vi "update execution error.vi"(8 "error in (no error)":errorcluster, 11 "Channel in":refnum<class "Channel.lvclass">) -> (0 "error out":errorcluster, 3 "Channel out":refnum<class "Channel.lvclass">)   [LabVIEW 2018, in "Channel.lvclass"]
doc: "Verify if there is an error in the error array of the camera class\n\nThis function will return true if there is any error or warning in the error array of the camera with a code different of 20002 or 0."
uses:
  Channel.lvclass
  Channel.lvclass/Channel.ctl
  Simulated_CCD_Camera/Simulated_CCD_Camera.lvclass/Simulated_CCD_Camera.ctl
  <vilib>/Utility/error.llb/Error Cluster From Error Code.vi
  <vilib>/ErrorRing/Error Ring.xnode
  Simulated_CCD_Camera/Simulated_CCD_Camera.lvclass
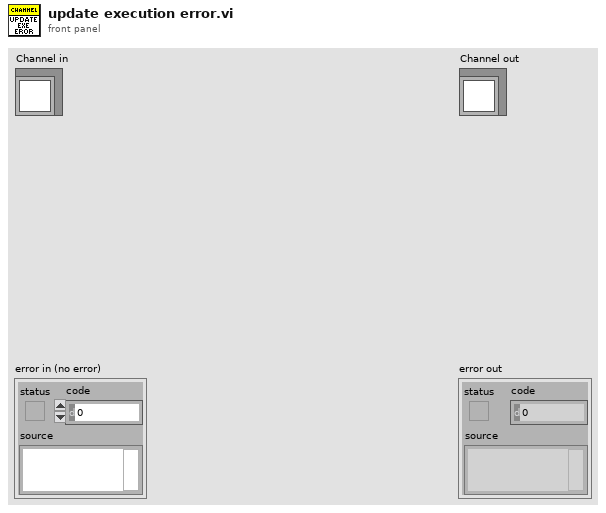
[diagram p1: front panel]
types:
  T1 = cluster{"CYCLES_DONE":u16, "LAST_IMAGE_NAME":string, "DISK_SPACE":u16, "FRAMES_DONE":u16, "CCD_STATUS":string, "CURRENT_TEMPERATURE":i16, "TEMPERATURE_STATUS":string, "FRAME_EXPOSURE_TIME":sgl, "ERROR":bool, "SERIAL_NUMBER":u16, "ACQUIRING":bool, "IMAGE_INDEX":u32, "SEQS_DONE":u16}
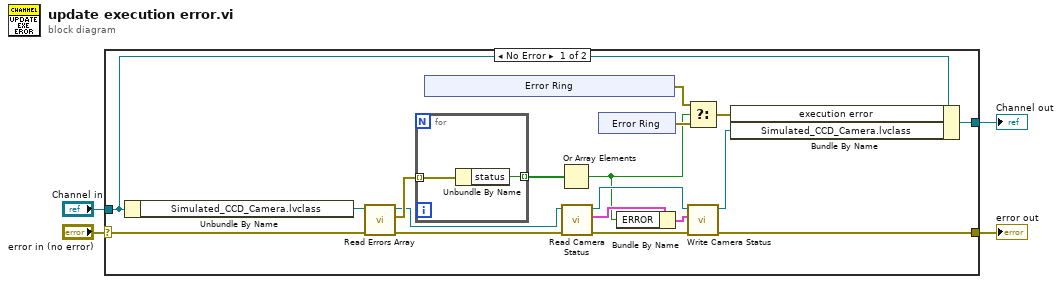
[diagram p0: block diagram]
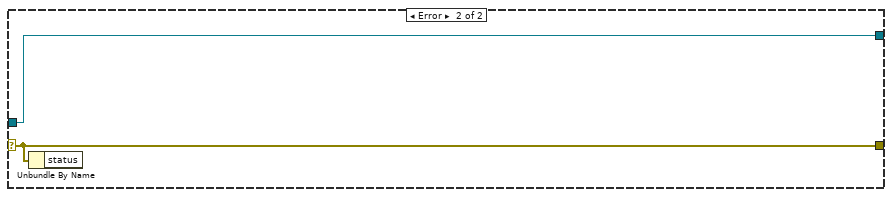
[diagram p2: hidden frame]
diagram:
  n1 = case shown="No Error" "error in (no error)" {
    selector: "error in (no error)" -> [w19 w31]
    tunnel: [w9 w31] -> w3
    tunnel: [w17 w32] -> w1
    tunnel: "Channel in" -> [w18 w32]
    frame No Error {
      n2 = Unbundle By Name(w18) -> ("Simulated_CCD_Camera.lvclass"=w22:refnum<class "Simulated_CCD_Camera.lvclass">)
      n3 = call "Read Errors Array.vi"("error in (no error)"=w19, "Simulated_CCD_Camera in"=w22) -> ("error out"=w13:errorcluster, "Errors array"=w21:errorcluster[], "Simulated_CCD_Camera out"=w12:refnum<class "Simulated_CCD_Camera.lvclass">)  [unwired: 7 in]
      n4 = for {
        tunnel: w21 -> [w30] mode=indexing
        tunnel: [w29] -> w20 mode=indexing
        n5 = Unbundle By Name(w30) -> ("status"=w29:bool)
      }
      n6 = xnode "Error Ring"() -> ("error out"=w16:errorcluster)
      n7 = Or Array Elements(Boolean array=w20) -> (logical OR=w5:bool)
      n8 = call "Read Camera Status.vi"("error in (no error)"=w13, "CCDCamera in"=w12) -> ("error out"=w8:errorcluster, "Camera Status"=w7:T1, "CCDCamera out"=w11:refnum<class "Simulated_CCD_Camera.lvclass">)  [unwired: 7 in]
      n9 = xnode "Error Ring"() -> ("error out"=w14:errorcluster)
      n10 = Bundle By Name(cluster=w7, "ERROR"=w5) -> (w6:T1)
      n11 = Select(t=w16, s=w5, f=w14) -> (s? t:f=w15:errorcluster)
      n12 = call "Write Camera Status.vi"("error in (no error)"=w8, "Camera Status"=w6, "CCDCamera in"=w11) -> ("error out"=w9:errorcluster, "CCDCamera out"=w10:refnum<class "Simulated_CCD_Camera.lvclass">)  [unwired: 7 in]
      n13 = Bundle By Name(cluster=w18, "execution error"=w15, "Simulated_CCD_Camera.lvclass"=w10) -> (w17:refnum<class "Channel.lvclass">)
    }
    frame Error {
      n14 = Unbundle By Name(w31) -> ()  [unwired: 1 out]
    }
  }
  "error out" <- w3
  "Channel out" <- w1
